vi "testMessage.vi"() -> (0 "error out":errorcluster)   [LabVIEW 2017, in "Assertion.Tests.lvlib" / "AssertTrue.lvlib"]
uses:
  AssertTrue.lvlib
  Assertion/Assertion.lvlib
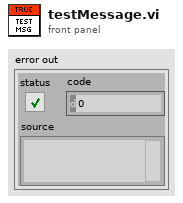
[diagram p1: front panel]
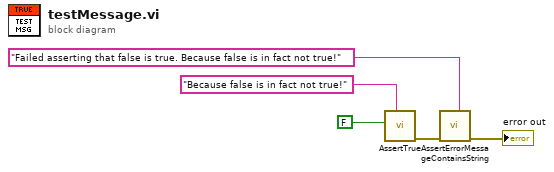
[diagram p0: block diagram]
diagram:
  n1 = call "AssertTrue.vi"("Message (\"\")"="Because false is in fact not true!" ("Message (\"\")"), "Condition"=FALSE) -> ("error out"=w4:errorcluster)  [unwired: 9 in]
  n2 = call "AssertErrorMessageContainsString.vi"("Expected"="Failed asserting that false is true. Because false is in fact not true!" ("y"), "error in (no error)"=w4) -> ("error out"=→"error out":errorcluster)  [unwired: 9 in]
